vi "EPad Sign Link.vi"(4 "Picture Subset":T1, 6 "OrgName":string, 7 "Name":string, 8 "e PadHeight":i32=100, 9 "ePad Width":i32=400, 10 "Filename":string, 11 "Path":path) -> (2 "Signature":picture, 3 "SignOK":bool)   [LabVIEW 2017]
uses:
  <vilib>/picture/picture.llb/imagedata.ctl
  <vilib>/Utility/miscctls.llb/LVBoundsTypeDef.ctl
panel:
  out "error out":errorcluster
  out "e":bool
  out "data":u8[](array[numeric])
  in  "ImageQuality":i32=200
  in  "image data":T2={"image type"=0, "image depth"=24, "image"=[], "mask"=[], "colors"=[], "Rectangle"={"left"=0, "top"=0, "right"=0, "bottom"=0}}
  in  "esCapture":refnum<k7>(container)
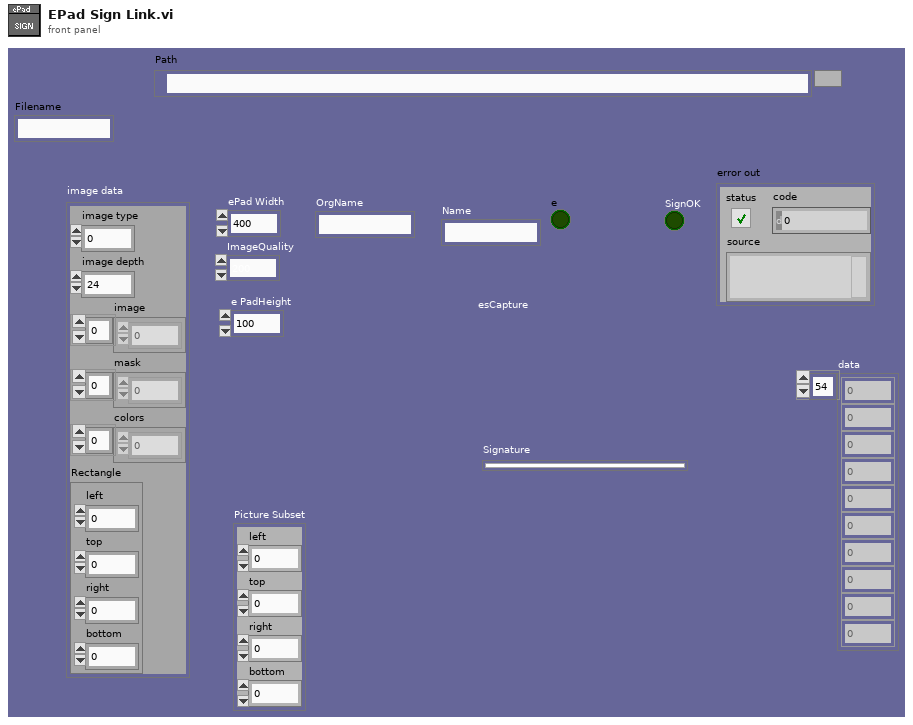
[diagram p1: front panel]
types:
  T1 = cluster{"left":i16, "top":i16, "right":i16, "bottom":i16}
  T2 = typedef "imagedata.ctl" = cluster{"image type":i32, "image depth":i32, "image":u8[], "mask":u8[], "colors":u32[], "Rectangle":cluster{"left":i16, "top":i16, "right":i16, "bottom":i16}}
  T3 = cluster{"Width":u16, "Style":enum32{"Solid", "Dash", "Dot", "DashDot", "DashDotDot"}}
  T4 = typedef "LVBoundsTypeDef.ctl" = cluster{"Width":u32, "Height":u32}
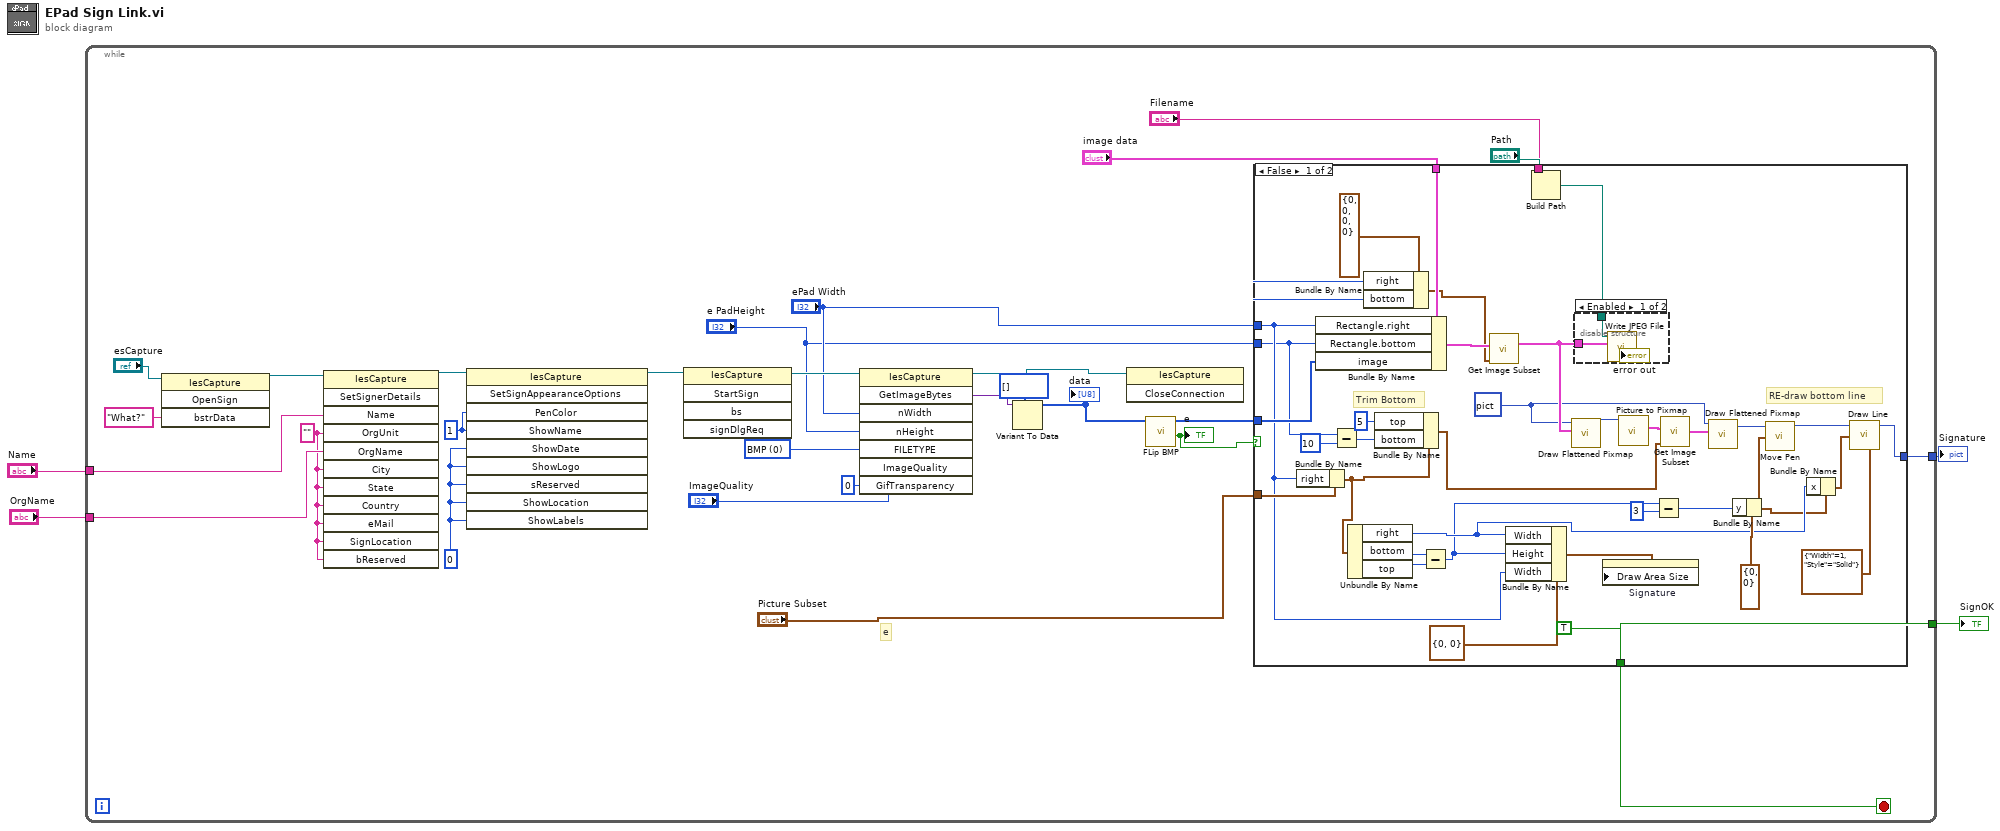
[diagram p0: block diagram]
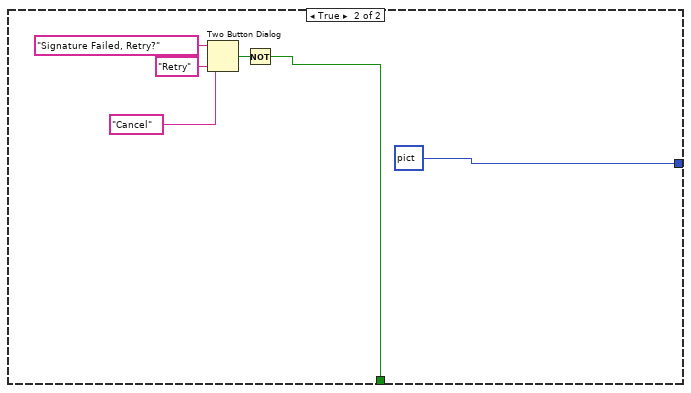
[diagram p3: hidden frame]
diagram:
  n1 = while {
    tunnel: "Name" -> [w19]
    tunnel: "OrgName" -> [w18]
    tunnel: [w14] -> w2
    tunnel: [w12] -> w1
    stop <- w12 stop-if-true
    w6 = i16 0 ("ShowName")
    w5 = i16 1 ("ShowName")
    w17 = "" ("OrgUnit")
    w30 = 0 items=["BMP", "JPEG", "GIF"] ("FILETYPE")
    # "e"
    n2 = invoke class="IesCapture" method="OpenSign"(reference="esCapture", "bstrData"="What?") -> (reference out=w20:refnum<k7>)  [unwired: 2 in, 3 out]
    n3 = invoke class="IesCapture" method="SetSignerDetails"(reference=w20, "Name"=w19, "OrgUnit"=w17, "OrgName"=w18, "City"=w17, "State"=w17, "Country"=w17, "eMail"=w17, "SignLocation"=w17, "bReserved"=w17) -> (reference out=w8:refnum<k7>)  [unwired: 2 in, 11 out]
    n4 = invoke class="IesCapture" method="SetSignAppearanceOptions"(reference=w8, "PenColor"=w5, "ShowName"=w5, "ShowDate"=w6, "ShowLogo"=w6, "sReserved"=w6, "ShowLocation"=w6, "ShowLabels"=w6) -> (reference out=w7:refnum<k7>)  [unwired: 2 in, 9 out]
    n5 = invoke class="IesCapture" method="StartSign"(reference=w7) -> (reference out=w16:refnum<k7>)  [unwired: 4 in, 4 out]
    n6 = invoke class="IesCapture" method="GetImageBytes"(reference=w16, "nWidth"="ePad Width", "nHeight"="e PadHeight", "FILETYPE"=w30, "ImageQuality"="ImageQuality", "GifTransparency"=0) -> (reference out=w13:refnum<k7>, "GetImageBytes"=w26:variant)  [unwired: 2 in, 6 out]
    n7 = Variant To Data(type=u8[] [], Variant=w26) -> (data=w22:u8[])  [unwired: 1 in, 1 out]
    "data" <- w22
    n8 = invoke class="IesCapture" method="CloseConnection"(reference=w13) -> ()  [unwired: 2 in, 3 out]
    n9 = call "FLip BMP.vi"("data"=w22) -> ("Blank Image"=w15:bool, "Array"=w21:u8[])  [unwired: 9 in]
    "e" <- w15
    n10 = case shown="False" w15 {
      tunnel: "image data" -> [w69 _]
      tunnel: "Path" -> [w68 _]
      tunnel: "Filename" -> [w67 _]
      tunnel: w21 -> [w61 _]
      tunnel: "ePad Width" -> [w51 _]
      tunnel: "e PadHeight" -> [w37 _]
      tunnel: [w42 picture data[5B] ("new picture")] -> w14
      tunnel: [TRUE w76] -> w12
      tunnel: "Picture Subset" -> [w53 _]
      frame False {
        w56 = picture data[5B] ("picture")
        # "RE-draw bottom line"
        # "Trim Bottom"
        n11 = Bundle By Name(cluster=w53, "right"=w51) -> (w38:T1)
        n12 = Bundle By Name(cluster=w69, "Rectangle.right"=w51, "Rectangle.bottom"=w37, "image"=w61) -> (w65:T2)
        n13 = Subtract(x=w37, y=10) -> (x-y=w35:i32)
        n14 = Unbundle By Name(w38) -> ("right"=w46:i16, "bottom"=w49:i16, "top"=w52:i16)
        n15 = Bundle By Name(cluster=T1 {"left"=0, "top"=0, "right"=0, "bottom"=0} ("subset rect"), "right"=w51, "bottom"=w37) -> (w62:T1)
        n16 = Bundle By Name(cluster=w38, "top"=i16 5, "bottom"=w35) -> (w33:T1)
        n17 = Subtract(x=w49, y=w52) -> (x-y=w40:i16)
        n18 = call <vilib>:"Get Image Subset.vi"("subset rect"=w62, "image data"=w65) -> ("image subset"=w64:T2)  [unwired: 4 in, 1 out]
        n19 = Bundle By Name(cluster=T4 {"Width"=0, "Height"=0} ("Draw Area Size"), "Width"=w46, "Height"=w40, "Width"=w51) -> (w55:T4)
        n20 = Build Path(base path=w68, name or relative path=w67) -> (appended path=w66:path)
        n21 = call <vilib>:"Draw Flattened Pixmap.vi"("image data"=w64, "picture"=w56) -> ("new picture"=w58:picture)  [unwired: 7 in]
        n22 = disable-structure shown="Enabled" {
          disable-tunnel: w64 -> [w72 _]
          disable-tunnel: w66 -> [w71 _]
          frame Enabled {
            n23 = call <vilib>:"Write JPEG File.vi"("image data"=w72, "path to JPEG file"=w71) -> ("error out"=→"error out":errorcluster)  [unwired: 8 in, 1 out]
          }
          frame Disabled {
          }
        }
        n24 = property on="Signature" class="Pict"("Draw Area Size"=w55) -> ()  [unwired: 2 in, 2 out]
        n25 = call <vilib>:"Picture to Pixmap.vi"("picture"=w58) -> ("image data"=w59:T2)  [unwired: 9 in, 1 out]
        n26 = Subtract(x=w40, y=i16 3) -> (x-y=w39:i16)
        n27 = call <vilib>:"Get Image Subset.vi"("subset rect"=w33, "image data"=w59) -> ("image subset"=w57:T2)  [unwired: 4 in, 1 out]
        n28 = call <vilib>:"Draw Flattened Pixmap.vi"("image data"=w57, "picture"=w56) -> ("new picture"=w50:picture)  [unwired: 7 in]
        n29 = Bundle By Name(cluster=cluster{"x":i16, "y":i16} {"x"=0, "y"=0} ("end point"), "y"=w39) -> (w45:cluster{"x":i16, "y":i16})
        n30 = call <vilib>:"Move Pen.vi"("new position"=w45, "picture"=w50) -> ("new picture"=w43:picture)  [unwired: 3 in]
        n31 = Bundle By Name(cluster=w45, "x"=w46) -> (w44:cluster{"x":i16, "y":i16})
        n32 = call <vilib>:"Draw Line.vi"("picture"=w43, "end point"=w44, "pen"=T3 {"Width"=1, "Style"=enum."Solid"}) -> ("new picture"=w42:picture)  [unwired: 6 in]
      }
      frame True {
        n33 = Two Button Dialog(message="Signature Failed, Retry?", 1:"Cancel" ("F button name (\"Cancel\")"), 2:"Retry" ("T button name (\"OK\")")) -> (T button?=w77:bool)
        n34 = Not(x=w77) -> (.not. x?=w76:bool)
      }
    }
  }
  "Signature" <- w2
  "SignOK" <- w1
